vi "Call The Create Error VI Creator.vi"(8 "error in":errorcluster, 10 "Library":refnum<class "Library.lvclass">, 11 "Project in":refnum<class "Project.lvclass">) -> (0 "error out":errorcluster, 1 "Cancel Out":bool, 2 "Item Tag":string, 3 "Project out":refnum<class "Project.lvclass">)   [LabVIEW 2020, in "Panther Dashboard.lvlib"]
uses:
  Panther Dashboard.lvlib
  Class/Library/Library.lvclass
  C:/GitClones/PantherDashboard/src/LabVIEW/Panther Dashboard/Class/LabVIEWItem/LabVIEWItem.lvclass
  Class/Project/Project.lvclass
  <vilib>/PantherLAB/Panther Constants and Errors/Libraries/ConstantErrorsMaker/Selection Info--cluster.ctl
  <vilib>/PantherLAB/Panther Constants and Errors/Libraries/ConstantErrorsMaker/Selection Type--enum.ctl
  Class/LabVIEWItem/LabVIEWItem.lvclass/LabVIEWItem.ctl
  Class/Library/Library.lvclass/Library.ctl
  Class/Project/Project.lvclass/Project.ctl
  Class/LabVIEWItem/Item Type--enum.ctl
  Class/VI/VI.lvclass
  Class/LabVIEWItem/Write Item Name.vi
  Class/LabVIEWItem/Write Item Description.vi
  Class/LabVIEWItem/Write Item Path.vi
  Class/LabVIEWItem/Write Item Type.vi
  Class/LabVIEWItem/Read Item Tag.vi
  Class/Library/Read Library Ref.vi
  Class/LabVIEWItem/Read Item Path.vi
  Class/Library/Read Type.vi
  Class/Project/Read Project Ref.vi
  Class/Project/Read Main App Inst Ref.vi
  <vilib>/PantherLAB/Panther Constants and Errors/Libraries/ConstantErrorsMaker/PantherLAB_lib_Panther_Constants_and_ErrorsConstantErrorsMaker.lvlib
  Class/LabVIEWItem/LabVIEWItem.lvclass
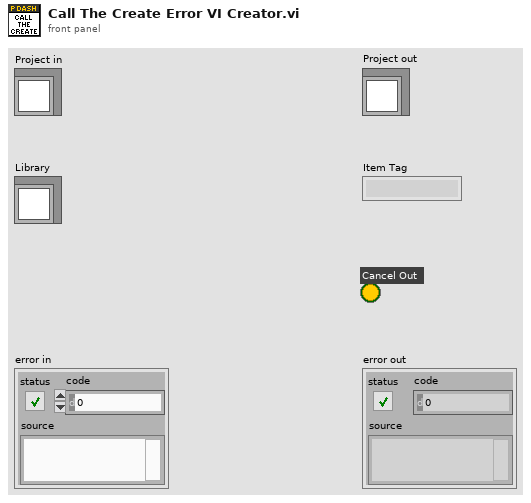
[diagram p1: front panel]
types:
  T1 = typedef "PantherLAB_lib_Panther_Constants_and_ErrorsConstantErrorsMaker.lvlib/Selection Info--cluster.ctl" = cluster{"Name":string, "Library Ref":refnum<vi>, "Application Instance":refnum<vi>, "Selection Owning Folder":path, "Selection Type":T2, "Project Reference":refnum<vi>, "LVClassLibrary Refnum":refnum<vi>}
  T2 = typedef "PantherLAB_lib_Panther_Constants_and_ErrorsConstantErrorsMaker.lvlib/Selection Type--enum.ctl" = enum16{"Project", "Library", "Class", "DQMH Singleton", "DQMH Cloneable"}
  T3 = typedef "Panther Dashboard.lvlib/Module type--enum.ctl" = enum16{"Singleton", "Cloneable"}
  T4 = typedef "Panther Dashboard.lvlib/LabVIEWItem.lvclass/Item Type--enum.ctl" = enum16{"Requests", "Broadcasts", "Request and Wait for Reply", "Round Trip", "» Public API VIs", "» Constant VIs", "» Error VIs", "Module", "Project", "No Drag Selection"}
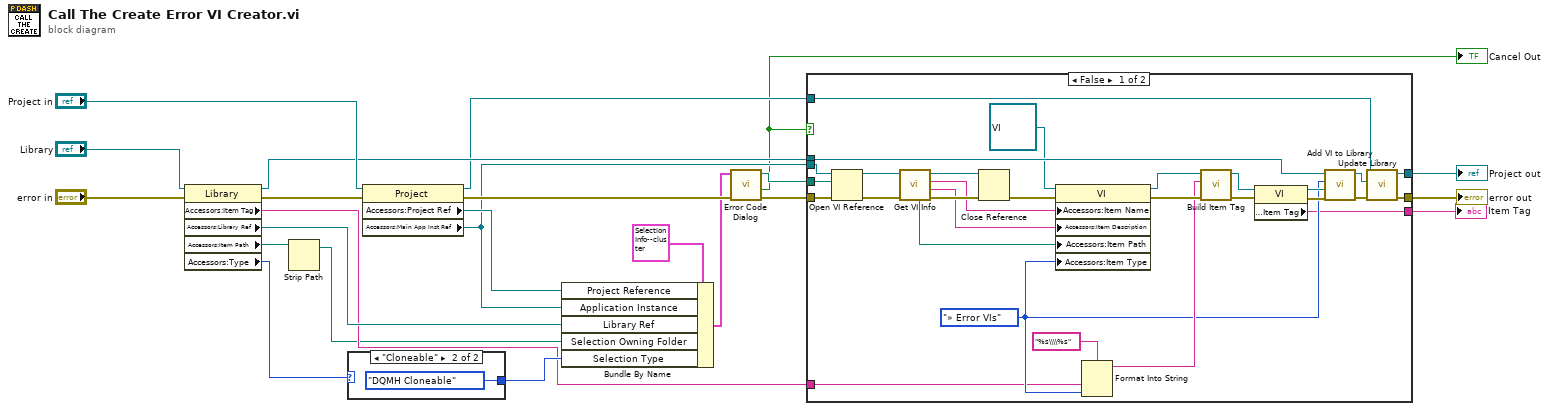
[diagram p0: block diagram]
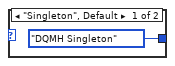
[diagram p3: hidden frame]
diagram:
  n1 = property class="Library"(reference="Library", error in="error in") -> (reference out=w12:refnum<class "Library.lvclass">, error out=w22:errorcluster, "Accessors:Item Tag"=w7:string, "Accessors:Library Ref"=w8:refnum<vi>, "Accessors:Item Path"=w16:path, "Accessors:Type"=w15:T3)
  n2 = Strip Path(path=w16) -> (stripped path=w1:path)  [unwired: 1 out]
  n3 = case shown="\"Cloneable\"" w15 {
    tunnel: [Selection_Type--enum."DQMH Singleton" ("Selection Type") Selection_Type--enum."DQMH Cloneable" ("Selection Type")] -> w14
    frame "Singleton", Default {
    }
    frame "Cloneable" {
    }
  }
  n4 = property class="Project"(reference="Project in", error in=w22) -> (reference out=w11:refnum<class "Project.lvclass">, error out=w21:errorcluster, "Accessors:Project Ref"=w13:refnum<vi>, "Accessors:Main App Inst Ref"=w9:refnum<vi>)
  n5 = Bundle By Name(cluster=T1 {"Name"="", "Library Ref"=refnum, "Application Instance"=refnum, "Selection Owning Folder"=path "", "Selection Type"=enum."Project", "Project Reference"=refnum, "LVClassLibrary Refnum"=refnum} ("Selection"), "Project Reference"=w13, "Application Instance"=w9, "Library Ref"=w8, "Selection Owning Folder"=w1, "Selection Type"=w14) -> (w3:T1)
  n6 = call <vilib>:"Error Code Dialog.vi"("error in"=w21, "Selection"=w3) -> ("error out"=w4:errorcluster, "Cancel Out"=w2:bool, "Error VI Path"=w5:path)  [unwired: 7 in]
  "Cancel Out" <- w2
  n7 = case shown="False" w2 {
    tunnel: [w51 w56] -> w20
    tunnel: w12 -> [w42 _]
    tunnel: w11 -> [w41 w57]
    tunnel: [w34 w57] -> w10
    tunnel: w9 -> [w33 _]
    tunnel: w7 -> [w29 w55]
    tunnel: [w28 w55] -> w6
    tunnel: w5 -> [w27 _]
    tunnel: w4 -> [w26 w56]
    frame False {
      w30 = Item_Type--enum."» Error VIs" ("VI Type")
      n8 = Open VI Reference(application reference (local)=w33, vi path=w27, error in (no error)=w26) -> (vi reference=w32:refnum<vi>, error out=w50:errorcluster)  [unwired: 3 in]
      n9 = call "Get VI Info.vi"("error in"=w50, "VI in"=w32) -> ("error out"=w54:errorcluster, "VI Description"=w36:string, "Plain Name"=w37:string, "VI out"=w31:refnum<vi>, "VI Path"=w35:path)  [unwired: 4 in, 1 out]
      n10 = Close Reference(reference=w31, error in (no error)=w54) -> (error out=w49:errorcluster)
      n11 = property class="VI"(reference=refnum<class "VI.lvclass"> refnum ("VI"), error in=w49, "Accessors:Item Name"=w37, "Accessors:Item Description"=w36, "Accessors:Item Path"=w35, "Accessors:Item Type"=w30) -> (reference out=w38:refnum<class "VI.lvclass">, error out=w48:errorcluster)
      n12 = Format Into String(format string="%s\\\\%s", w29, w30) -> (resulting string=w45:string)  [unwired: 2 in, 1 out]
      n13 = call "Build Item Tag.vi"("error in"=w48, "Parent Tag"=w45, "LabVIEWItem in"=w38) -> ("error out"=w47:errorcluster, "LabVIEWItem out"=w46:refnum<class "VI.lvclass">)  [unwired: 7 in]
      n14 = property class="VI"(reference=w46, error in=w47) -> (reference out=w40:refnum<class "VI.lvclass">, error out=w53:errorcluster, "Accessors:Item Tag"=w28:string)
      n15 = call "Add VI to Library.vi"("error in"=w53, "VI"=w40, "VI Type"=w30, "Library in"=w42) -> ("error out"=w52:errorcluster, "Library out"=w43:refnum<class "Library.lvclass">)  [unwired: 6 in]
      n16 = call "Update Library.vi"("error in"=w52, "Library"=w43, "Project in"=w41) -> ("error out"=w51:errorcluster, "Project out"=w34:refnum<class "Project.lvclass">)  [unwired: 7 in]
    }
    frame True {
    }
  }
  "error out" <- w20
  "Project out" <- w10
  "Item Tag" <- w6
